vi "Installment of the Project in LabVIEW.vi"() -> ()   [LabVIEW 2020]
panel:
  in  "Table Control":string[][](table)
  in  "VISA resource name":refnum<visa-resource-name>
  out "gas Chart 2":dbl(graph)
  out "Temperature Chart":dbl(graph)
  out "?":dbl(knob) scale=0.0..100.0
  out "Temperature":dbl(slide) scale=0.0..100.0
  # "Humidity"
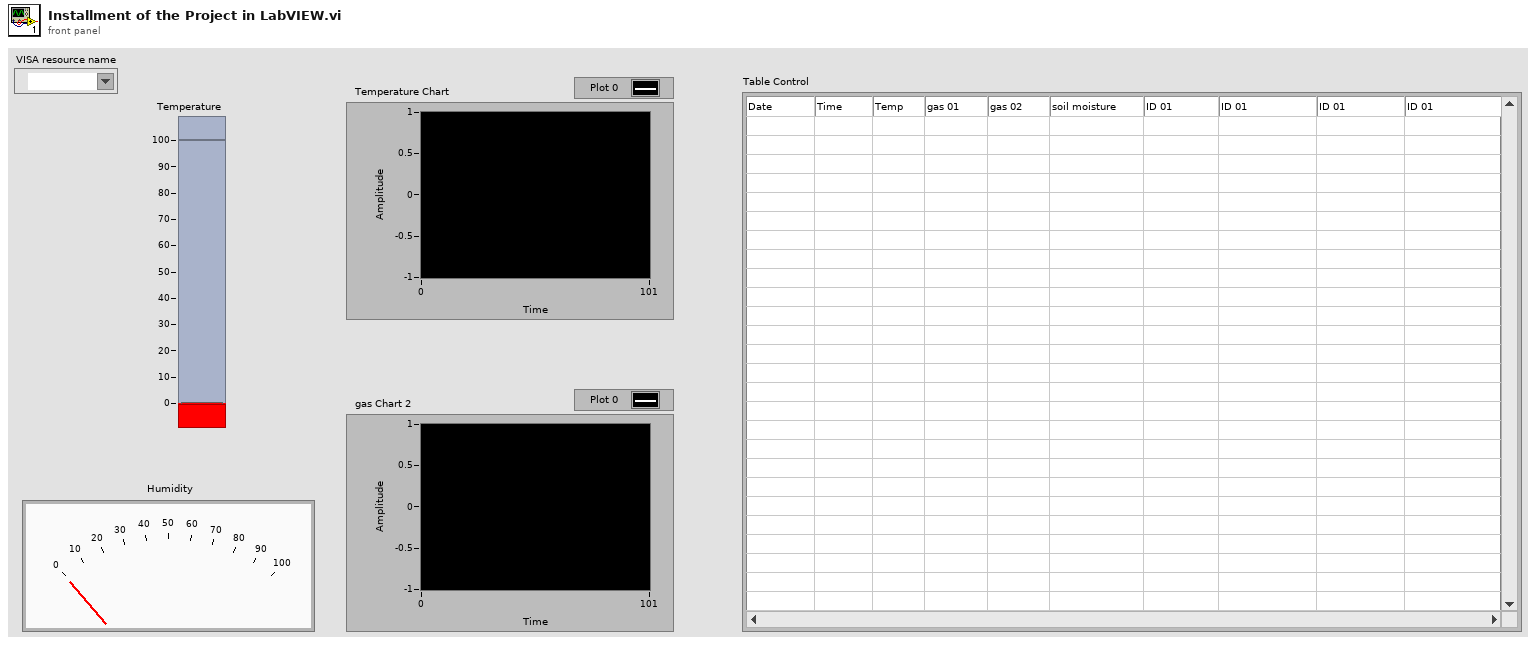
[diagram p1: front panel]
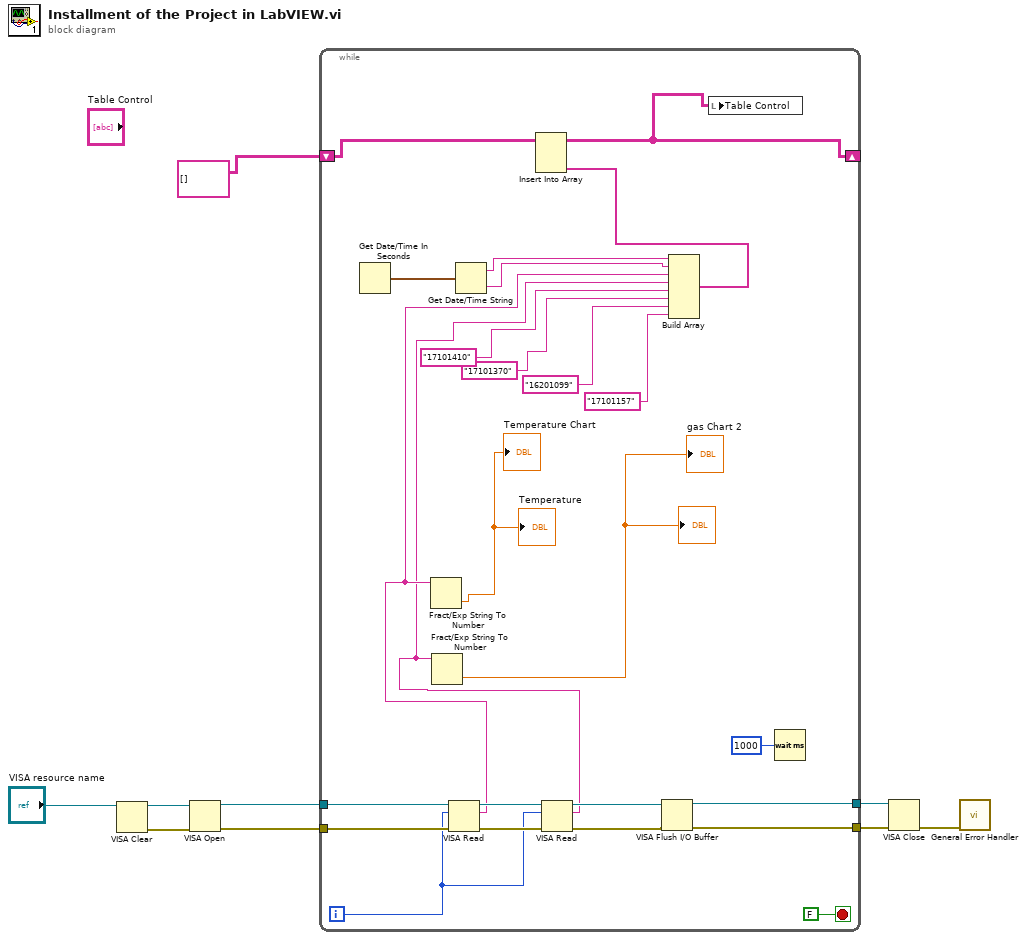
[diagram p0: block diagram]
diagram:
  n1 = VISA Clear(VISA resource name="VISA resource name") -> (VISA resource name out=w4:refnum<visa-resource-name>, error out=w3:errorcluster)  [unwired: 1 in]
  n2 = VISA Open(error in (no error)=w3, VISA resource name=w4) -> (VISA resource name=w9:refnum<visa-resource-name>, error out=w8:errorcluster)  [unwired: 3 in]
  n3 = while {
    tunnel: w9 -> [w34]
    tunnel: w8 -> [w33]
    tunnel: [w28] -> w7
    tunnel: [w27] -> w6
    shift-right: [w18] -> _
    shift-left: string[][] [] -> [w19]
    i -> [w26]
    stop <- FALSE stop-if-true
    n4 = Get Date/Time In Seconds() -> (seconds since 1Jan1904=w22:timestamp)
    n5 = VISA Read(VISA resource name=w34, byte count=w26, error in (no error)=w33) -> (VISA resource name out=w32:refnum<visa-resource-name>, read buffer=w15:string, error out=w31:errorcluster)  [unwired: 1 out]
    n6 = Fract/Exp String To Number(string=w15) -> (number=→"Temperature Chart" →"Temperature":dbl)  [unwired: 3 in, 1 out]
    n7 = Get Date/Time String(seconds (now)=w22) -> (date string=w17:string, time string=w16:string)  [unwired: 2 in]
    n8 = VISA Read(VISA resource name=w32, byte count=w26, error in (no error)=w31) -> (VISA resource name out=w30:refnum<visa-resource-name>, read buffer=w14:string, error out=w29:errorcluster)  [unwired: 1 out]
    n9 = Fract/Exp String To Number(string=w14) -> (number=→"gas Chart 2" →"?":dbl)  [unwired: 3 in, 1 out]
    n10 = VISA Flush I/O Buffer(VISA resource name=w30, error in (no error)=w29) -> (VISA resource name out=w27:refnum<visa-resource-name>, error out=w28:errorcluster)  [unwired: 1 in]
    n11 = Build Array(w17, w16, w15, w14, "17101410" ("element"), "17101370" ("element"), "16201099" ("element"), "17101157" ("element")) -> (w20:string[])
    n12 = Insert Into Array(array=w19, new element=w20) -> (w18:string[][])  [unwired: 2 in]
    n13 = local write "Table Control"(w18) -> ()
    n14 = Wait (ms)(milliseconds to wait=u32 1000 ("millisecond timer value")) -> ()  [unwired: 1 out]
  }
  n15 = VISA Close(VISA resource name=w6, error in (no error)=w7) -> (error out=w5:errorcluster)
  n16 = call <vilib>:"General Error Handler.vi"("error in (no error)"=w5) -> ()  [unwired: 10 in, 5 out]
